vi "X_Stage.vi"(11 "X-Coordinate":dbl) -> ()   [LabVIEW 2013]
panel:
  out "Current X Position":sgl
  in  "MG17Motor 3":refnum<k7>(container)
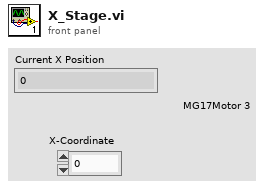
[diagram p1: front panel]
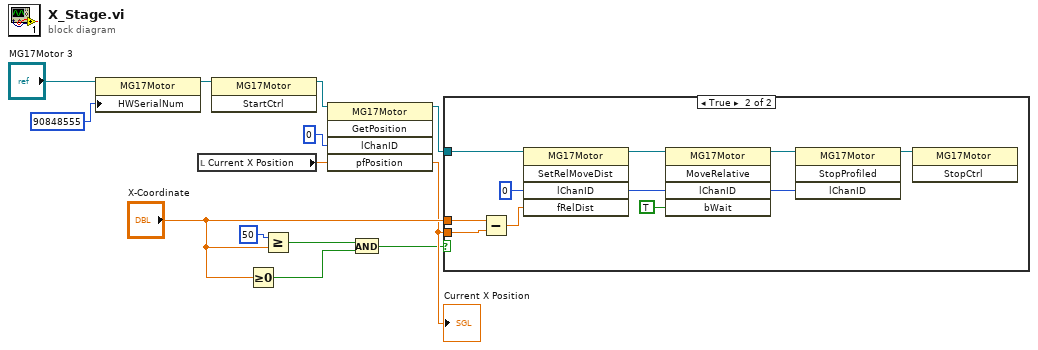
[diagram p0: block diagram]
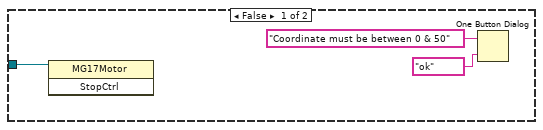
[diagram p2: hidden frame]
diagram:
  n1 = property class="MG17Motor"(reference="MG17Motor 3", "HWSerialNum"=90848555 ("lChanID")) -> (reference out=w12:refnum<k7>)  [unwired: 1 in, 1 out]
  n2 = local read "Current X Position"() -> (w9:sgl)
  n3 = invoke class="MG17Motor" method="StartCtrl"(reference=w12) -> (reference out=w10:refnum<k7>)  [unwired: 2 in, 2 out]
  n4 = Greater Or Equal To 0?(x="X-Coordinate") -> (x >= 0?=w8:bool)
  n5 = Greater Or Equal?(x=50, y="X-Coordinate") -> (x >= y?=w7:bool)
  n6 = invoke class="MG17Motor" method="GetPosition"(reference=w10, "lChanID"=0, "pfPosition"=w9) -> (reference out=w2:refnum<k7>, "pfPosition"=w4:sgl)  [unwired: 2 in, 3 out]
  "Current X Position" <- w4
  n7 = And(x=w7, y=w8) -> (x .and. y?=w3:bool)
  n8 = case shown="True" w3 {
    tunnel: "X-Coordinate" -> [_ w18]
    tunnel: w4 -> [_ w17]
    tunnel: w2 -> [w16 w19]
    frame False {
      n9 = invoke class="MG17Motor" method="StopCtrl"(reference=w16) -> ()  [unwired: 2 in, 3 out]
      n10 = One Button Dialog(message="Coordinate must be between 0 & 50", button name ("OK")="ok") -> ()  [unwired: 1 out]
    }
    frame True {
      n11 = Subtract(x=w18, y=w17) -> (x-y=w20:dbl)
      n12 = invoke class="MG17Motor" method="SetRelMoveDist"(reference=w19, "lChanID"=0, "fRelDist"=w20) -> (reference out=w23:refnum<k7>, "lChanID"=w24:i32)  [unwired: 2 in, 3 out]
      n13 = invoke class="MG17Motor" method="MoveRelative"(reference=w23, "lChanID"=w24, "bWait"=TRUE) -> (reference out=w25:refnum<k7>, "lChanID"=w26:i32)  [unwired: 2 in, 3 out]
      n14 = invoke class="MG17Motor" method="StopProfiled"(reference=w25, "lChanID"=w26) -> (reference out=w27:refnum<k7>)  [unwired: 2 in, 3 out]
      n15 = invoke class="MG17Motor" method="StopCtrl"(reference=w27) -> ()  [unwired: 2 in, 3 out]
    }
  }
